vi "mlink_dio_read.vi"(8 "error in (no error)":errorcluster, 10 "pin":u8, 11 "connection ID":i32=-1) -> (0 "error out":errorcluster, 2 "state":bool, 3 "connection ID out":i32)   [LabVIEW 2009, in "MicroDAQ.lvlib" / "mlink.lvlib"]
doc: "This function reads DIO channel state. The function read channel and stores its state in \nvariable pointed by state."
uses:
  <instrlib>/MicroDAQ/Mlink library wraper/mlink.lvlib
  <instrlib>/MicroDAQ/MLink32.dll
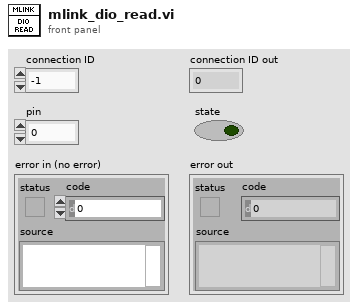
[diagram p1: front panel]
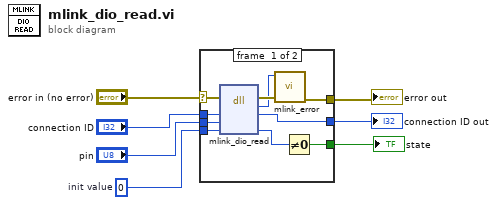
[diagram p0: block diagram]
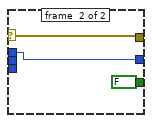
[diagram p2: hidden frame]
diagram:
  w5 = u8 0  # init value
  n1 = case shown="No Error" "error in (no error)" {
    selector: "error in (no error)" -> [w14 w20]
    tunnel: "connection ID" -> [w17 w19]
    tunnel: [w16 w19] -> w6
    tunnel: w5 -> [w15 _]
    tunnel: [w13 FALSE] -> w3
    tunnel: "pin" -> [w11 _]
    tunnel: [w8 w20] -> w1
    frame #0 {
      n2 = dll-call lib="C:/Program Files (x86)/National Instruments/LabVIEW 2009/instr.lib/MicroDAQ/MLink32.dll" fn="mlink_dio_read"(error in=w14, "connection ID"=w17, "pin"=w11, "value"=w15) -> (error out=w10:errorcluster, "return type"=w9:i32, "connection ID"=w16:i32, "value"=w12:u8)  [unwired: 3 in, 1 out]
      n3 = call <instrlib>:"mlink_error.vi"("error in (no error)"=w10, "error code"=w9) -> ("error out"=w8:errorcluster)  [unwired: 9 in]
      n4 = Not Equal To 0?(x=w12) -> (x != 0?=w13:bool)
    }
    frame #1 {
    }
  }
  "connection ID out" <- w6
  "error out" <- w1
  "state" <- w3
